vi "Practica 9.vi"() -> ()   [LabVIEW 2014]
panel:
  out "Vas requeridos\n por las pc 5":dbl
  out "Vas de las \ncomputadoras 5":dbl
  in  "CORRIENTES \nDE LAS COMPUTADORAS Amperes 5":dbl
  in  "NUM DE COMPUTADORAS 5":dbl
  in  "Voltaje en 220 WAC 5":dbl
  in  "Voltage 120AC 6":dbl
  out "Vas requeridos\n por las pc 4":dbl
  out "Vas de las \ncomputadoras 4":dbl
  in  "CORRIENTES \nDE LAS COMPUTADORAS Amperes 4":dbl
  in  "NUM DE COMPUTADORAS 4":dbl
  in  "Voltaje en 220 WAC 4":dbl
  in  "Voltage 120AC 5":dbl
  out "Vas requeridos\n por las pc 3":dbl
  out "Vas de las \ncomputadoras 3":dbl
  in  "CORRIENTES \nDE LAS COMPUTADORAS Amperes 3":dbl
  in  "NUM DE COMPUTADORAS 3":dbl
  in  "Voltaje en 220 WAC 3":dbl
  in  "Voltage 120AC 4":dbl
  out "Vas requeridos\n por las pc 2":dbl
  out "Vas de las \ncomputadoras 2":dbl
  in  "CORRIENTES \nDE LAS COMPUTADORAS Amperes 2":dbl
  in  "NUM DE COMPUTADORAS 2":dbl
  in  "Voltaje en 220 WAC 2":dbl
  in  "Voltage 120AC 3":dbl
  out "Vas requeridos\n por las pc":dbl
  out "Vas de las \ncomputadoras":dbl
  in  "CORRIENTES \nDE LAS COMPUTADORAS Amperes":dbl
  in  "NUM DE COMPUTADORAS":dbl
  in  "Voltaje en 220 WAC":dbl
  in  "Voltage 120AC":dbl
  # "Servidores"
  # "Modems"
  # "Switches"
  # "Microcomputadoras"
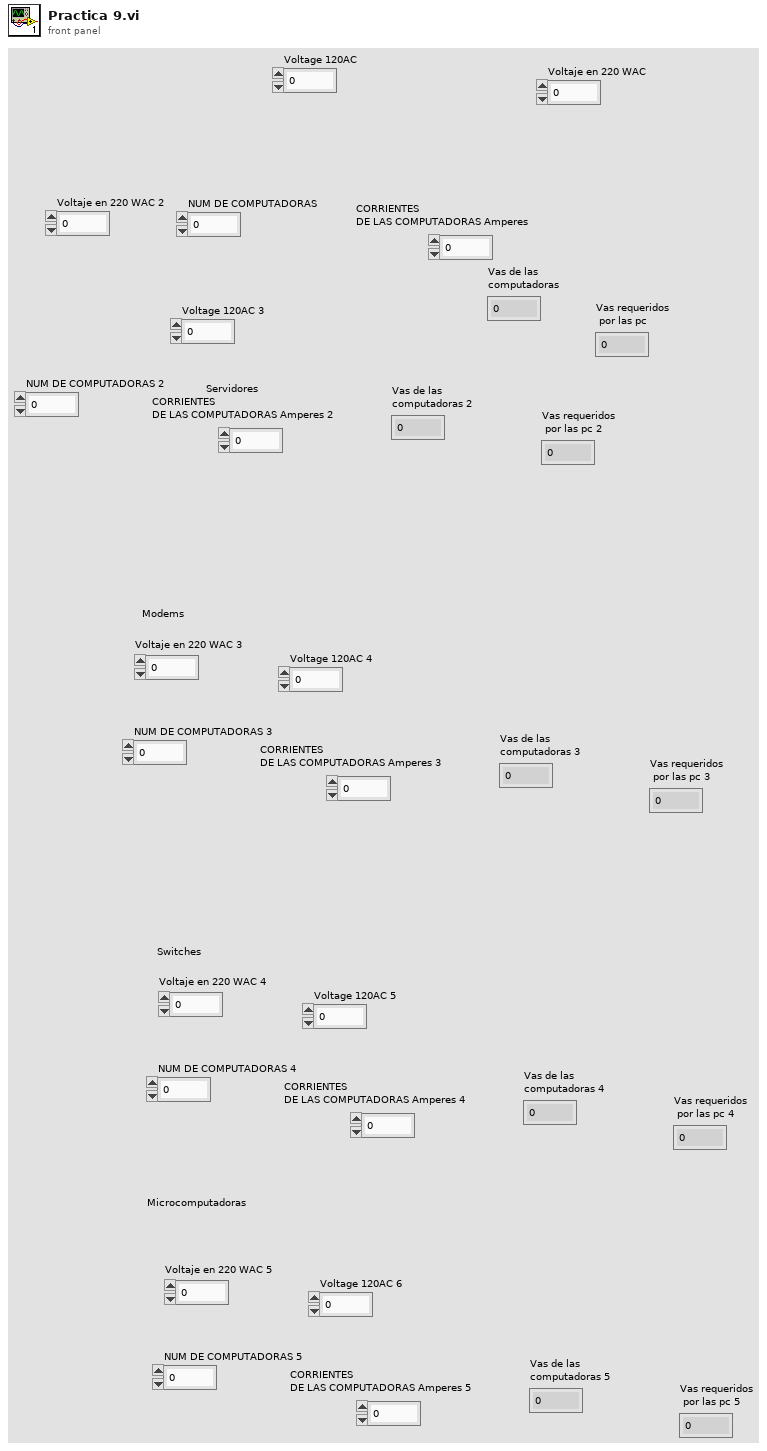
[diagram p1: front panel]
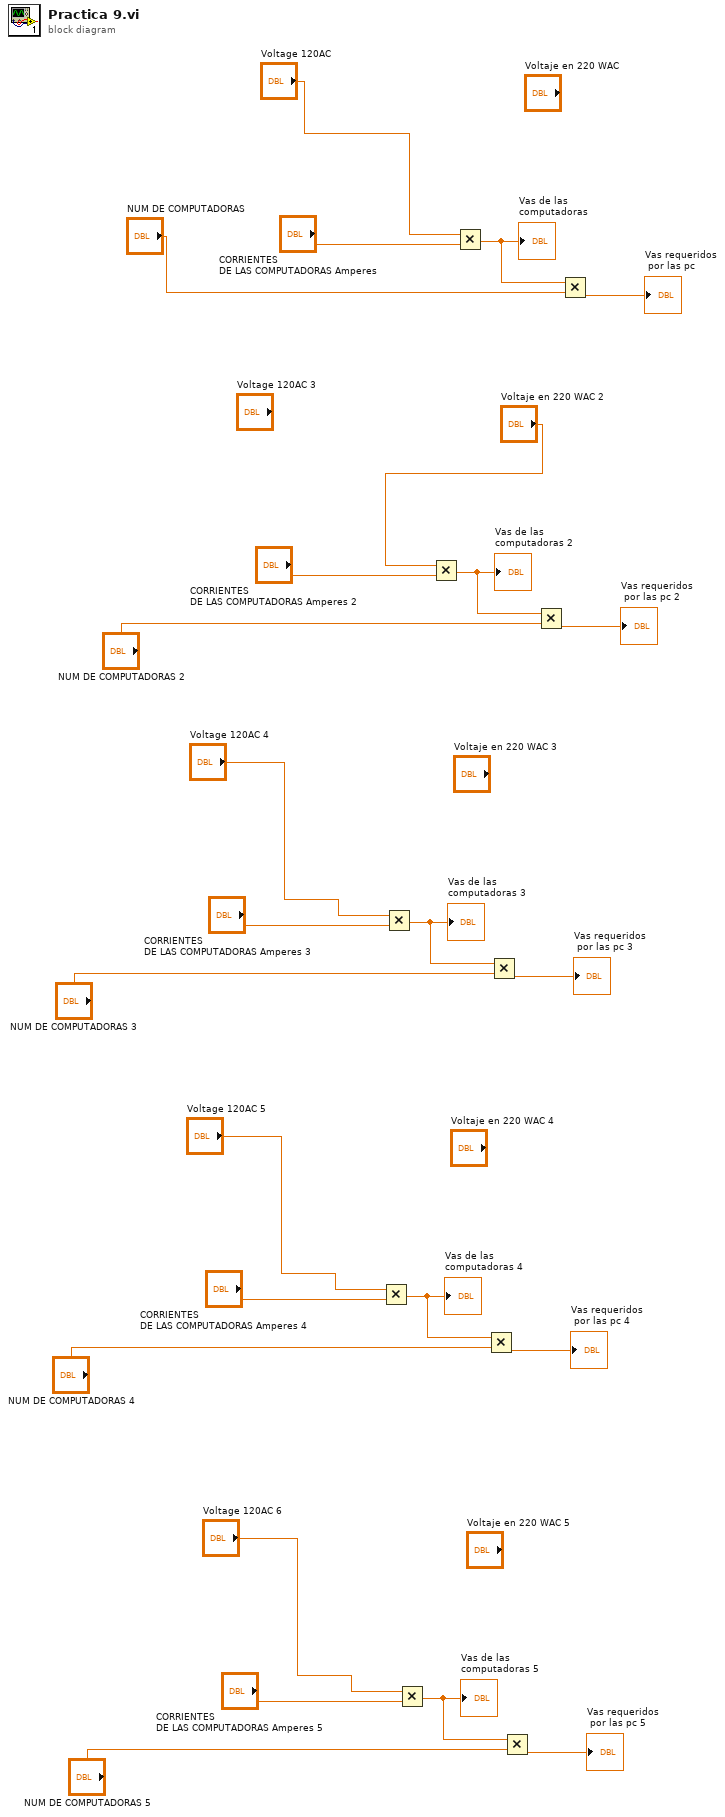
[diagram p0: block diagram]
diagram:
  n1 = Multiply(x="Voltage 120AC 5", y="CORRIENTES \nDE LAS COMPUTADORAS Amperes 4") -> (x*y=w7:dbl)
  "Vas de las \ncomputadoras 4" <- w7
  n2 = Multiply(x="Voltage 120AC 4", y="CORRIENTES \nDE LAS COMPUTADORAS Amperes 3") -> (x*y=w12:dbl)
  "Vas de las \ncomputadoras 3" <- w12
  n3 = Multiply(x="Voltage 120AC 6", y="CORRIENTES \nDE LAS COMPUTADORAS Amperes 5") -> (x*y=w2:dbl)
  "Vas de las \ncomputadoras 5" <- w2
  n4 = Multiply(x="Voltaje en 220 WAC 2", y="CORRIENTES \nDE LAS COMPUTADORAS Amperes 2") -> (x*y=w17:dbl)
  "Vas de las \ncomputadoras 2" <- w17
  n5 = Multiply(x="Voltage 120AC", y="CORRIENTES \nDE LAS COMPUTADORAS Amperes") -> (x*y=w21:dbl)
  "Vas de las \ncomputadoras" <- w21
  n6 = Multiply(x=w7, y="NUM DE COMPUTADORAS 4") -> (x*y=→"Vas requeridos\n por las pc 4":dbl)
  n7 = Multiply(x=w12, y="NUM DE COMPUTADORAS 3") -> (x*y=→"Vas requeridos\n por las pc 3":dbl)
  n8 = Multiply(x=w2, y="NUM DE COMPUTADORAS 5") -> (x*y=→"Vas requeridos\n por las pc 5":dbl)
  n9 = Multiply(x=w17, y="NUM DE COMPUTADORAS 2") -> (x*y=→"Vas requeridos\n por las pc 2":dbl)
  n10 = Multiply(x=w21, y="NUM DE COMPUTADORAS") -> (x*y=→"Vas requeridos\n por las pc":dbl)
